vi "PRAT Macro Get Power Data.vi"(8 "Error In":errorcluster, 11 "all rows":string[][](array[string])) -> (0 "Error Out":errorcluster, 1 "max value":dbl, 2 "standard deviation":dbl format="%0.2f", 3 "mean":dbl format="%0.2f", 4 "min value":dbl, 5 "DBL":dbl[](array[numeric]))   [LabVIEW 2016]
uses:
  <vilib>/Analysis/NI_AALBase.lvlib
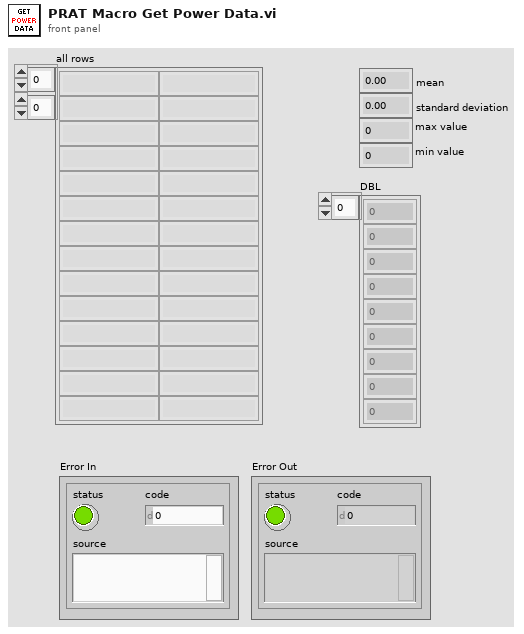
[diagram p1: front panel]
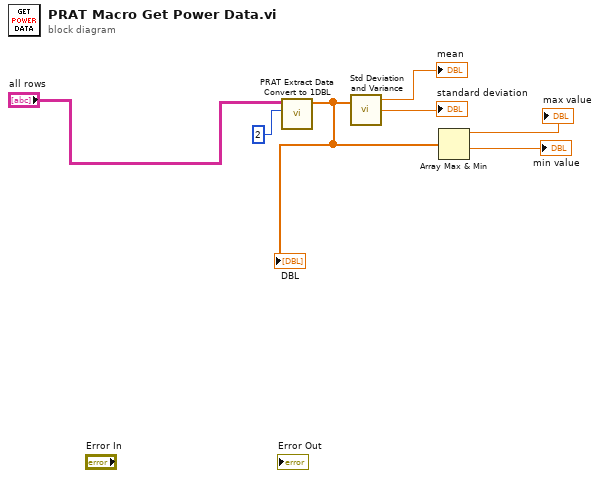
[diagram p0: block diagram]
diagram:
  n1 = call "PRAT Extract Data Convert to 1DBL.vi"("Extract Column"=2, "Full Cycle Data"="all rows") -> ("DBL"=w7:dbl[])  [unwired: 8 in, 1 out]
  "DBL" <- w7
  n2 = call <vilib>:"Std Deviation and Variance.vi"("X"=w7) -> ("mean"=→"mean":dbl, "standard deviation"=→"standard deviation":dbl)  [unwired: 1 in, 1 out]
  n3 = Array Max & Min(array=w7) -> (max value=→"max value":dbl, min value=→"min value":dbl)  [unwired: 2 out]
